vi "Cull and Group Vertical.vi"(9 "Score Cutoff":dbl=50.0, 10 "Sorted Data":dbl[][](array[numeric])) -> (0 "Rect":T1, 1 "Top Score":dbl, 3 "Center":cluster{"X":dbl, "Y":dbl}, 4 "Line":cluster{dbl, dbl, dbl, dbl})   [LabVIEW 2016]
doc: "Examine the particle measurements to find the most likely pair that make up the target. This mostly compares the edges of the bounding boxes. It then returns information about the overall target, notably the rectangle sourrounding the particles, the vertical line that bisects the target, and the center of the top particle."
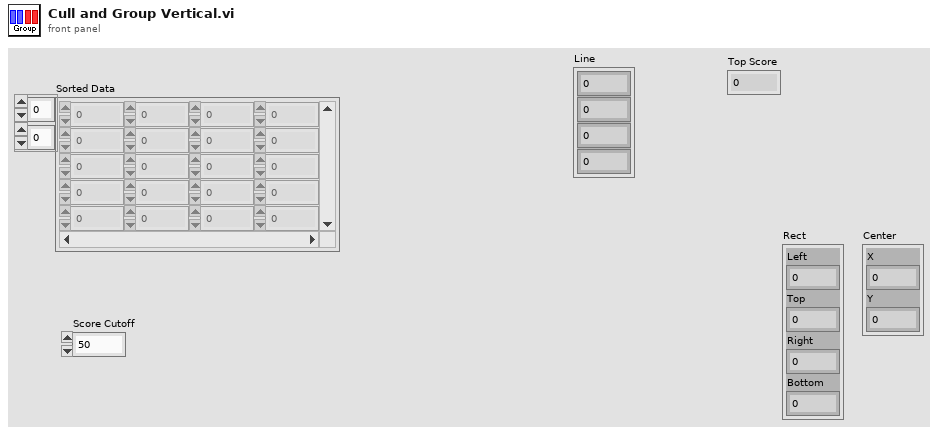
[diagram p1: front panel]
types:
  T1 = cluster{"Left":dbl, "Top":dbl, "Right":dbl, "Bottom":dbl}
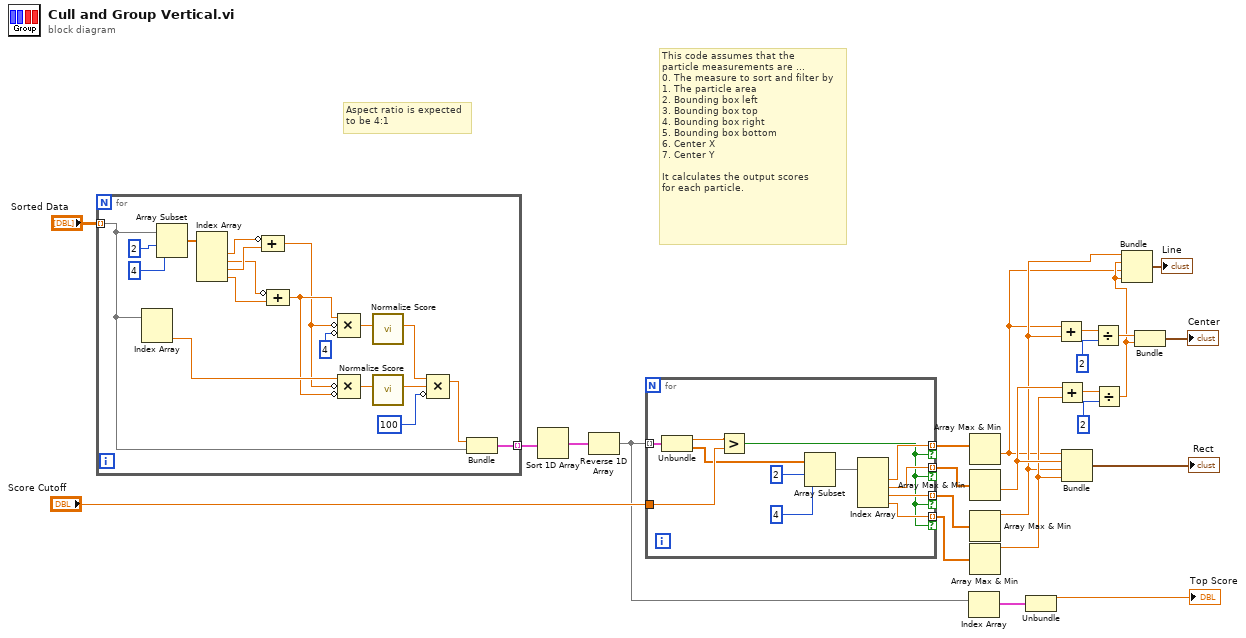
[diagram p0: block diagram]
diagram:
  # "Aspect ratio is expected\nto be 4:1"
  # "This code assumes that the\nparticle measurements are ...\n0. The measure to sort and filter by\n1. The particle area\n2. Bounding box left\n3. Bounding box top\n4. Bounding box right\n5. Bounding box bottom\n6. Center X\n7. Center Y\n\nIt calculates the output scores\nfor each particle."
  n1 = for {
    tunnel: "Sorted Data" -> [w28] mode=indexing
    tunnel: [w26] -> w23 mode=indexing
    n2 = Index Array(array=w28) -> (element #2=w34:dbl)  [unwired: 2 in, 1 out]
    n3 = Array Subset(array=w28, index=2, length=4) -> (w41:dbl[])
    n4 = Index Array(array=w41) -> (element #1=w39:dbl, element #2=w37:dbl, element #3=w40:dbl, element #4=w38:dbl)  [unwired: 4 in]
    n5 = Compound Arithmetic op=ADD(invert w39, w40) -> (w25:dbl)
    n6 = Compound Arithmetic op=ADD(invert w37, w38) -> (w33:dbl)
    n7 = Compound Arithmetic op=MULTIPLY(w33, invert w25, invert 4 ("length")) -> (w35:dbl)
    n8 = Compound Arithmetic op=MULTIPLY(w34, invert w25, invert w33) -> (w32:dbl)
    n9 = call "Normalize Score.vi"("Value"=w35) -> ("Score"=w31:dbl)  [unwired: 10 in]
    n10 = call "Normalize Score.vi"("Value"=w32) -> ("Score"=w30:dbl)  [unwired: 10 in]
    n11 = Compound Arithmetic op=MULTIPLY(w31, w30, invert 100 ("length")) -> (w27:dbl)
    n12 = Bundle(w27, "Sorted Data"=w28) -> (w26:cluster{dbl, "Sorted Data":dbl[]})  [unwired: 1 in]
  }
  n13 = Sort 1D Array(array=w23) -> (sorted array=w16:cluster{dbl, "Sorted Data":dbl[]}[])
  n14 = Reverse 1D Array(array=w16) -> (reversed array=w13:cluster{dbl, "Sorted Data":dbl[]}[])
  n15 = for {
    tunnel: w13 -> [w55] mode=indexing
    tunnel: "Score Cutoff" -> [w53]
    tunnel: [w48] -> w21 mode=indexing if=w44
    tunnel: [w47] -> w20 mode=indexing if=w44
    tunnel: [w46] -> w19 mode=indexing if=w44
    tunnel: [w45] -> w18 mode=indexing if=w44
    n16 = Unbundle(w55) -> (w54:dbl, "Sorted Data"=w49:dbl[])
    n17 = Greater?(x=w54, y=w53) -> (0:w44:bool)
    n18 = Array Subset(array=w49, index=2, length=4) -> (w52:dbl[])
    n19 = Index Array(array=w52) -> (element #1=w48:dbl, element #2=w47:dbl, element #3=w46:dbl, element #4=w45:dbl)  [unwired: 4 in]
  }
  n20 = Index Array(array=w13) -> (element=w15:cluster{dbl, "Sorted Data":dbl[]})  [unwired: 1 in]
  n21 = Array Max & Min(array=w21) -> (min value=w2:dbl)  [unwired: 3 out]
  n22 = Array Max & Min(array=w20) -> (min value=w6:dbl)  [unwired: 3 out]
  n23 = Array Max & Min(array=w19) -> (max value=w3:dbl)  [unwired: 3 out]
  n24 = Array Max & Min(array=w18) -> (max value=w5:dbl)  [unwired: 3 out]
  n25 = Unbundle(w15) -> (→"Top Score":dbl)  [unwired: 1 out]
  n26 = Add(x=w2, y=w3) -> (x+y=w11:dbl)
  n27 = Add(x=w6, y=w5) -> (x+y=w10:dbl)
  n28 = Bundle(w2, w6, w3, w5) -> (→"Rect":cluster{dbl, dbl, dbl, dbl})  [unwired: 1 in]
  n29 = Divide(x=w11, y=2 ("index")) -> (x/y=w7:dbl)
  n30 = Divide(x=w10, y=2 ("index")) -> (x/y=w4:dbl)
  n31 = Bundle(w3, w4, w2, w4) -> (→"Line":cluster{dbl, dbl, dbl, dbl})  [unwired: 1 in]
  n32 = Bundle(w7, w4) -> (→"Center":cluster{dbl, dbl})  [unwired: 1 in]
